vi "Teleop.vi"(10 "Match Info":T1={"Autonomous Elapsed Seconds"=0.0, "TeleOp Elapsed Seconds"=0.0, "Disabled Elapsed Seconds"=0.0, "Visited Autonomous"=FALSE, "Visited TeleOp"=FALSE, "Visited Disabled"=FALSE, "Autonomous Settings"={"Autonomous Style"=enum."Independent", "VI Refnum"=refnum}}, 11 "Call Context":T2) -> ()   [LabVIEW 2014]
doc: "This VI is called for each TeleOp packet received from the DS where the robot is not disabled. It is often used to read from the joysticks and update I/O or to update setpoints for timed control loops. It should complete and return within 20 milliseconds or it may miss DS packets."
uses:
  <vilib>/Rock Robotics/WPI/DriverStation/WPI_DriverStationDerivedRobotMode.ctl
  <vilib>/Rock Robotics/WPI/DriverStation/WPI_DriverStationMatch Info.ctl
  <vilib>/Rock Robotics/WPI/Relay/WPI_RelayValue.ctl
  Robot Global Data.vi
  <vilib>/Rock Robotics/WPI/RobotDrive/WPI_RobotDriveGetSetRefNum.vi
  <vilib>/Rock Robotics/WPI/Joystick/WPI_JoystickGetSetRefNum.vi
  <vilib>/Rock Robotics/WPI/Solenoid/WPI_SolenoidValue.ctl
  <vilib>/Rock Robotics/WPI/Solenoid/WPI_SolenoidSetEnum.vi
panel:
  out "Numeric 1":dbl(slide) scale=0.0..100.0
  out "Boolean 2":bool
  out "Boolean 1":bool
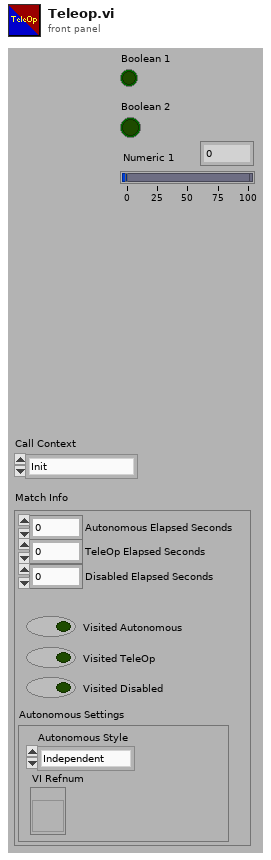
[diagram p1: front panel]
types:
  T1 = typedef "WPI_DriverStationMatch Info.ctl" = cluster{"Autonomous Elapsed Seconds":dbl, "TeleOp Elapsed Seconds":dbl, "Disabled Elapsed Seconds":dbl, "Visited Autonomous":bool, "Visited TeleOp":bool, "Visited Disabled":bool, "Autonomous Settings":cluster{"Autonomous Style":enum16{"Iterative", "Independent"}, "VI Refnum":refnum<vi>}}
  T2 = typedef "WPI_DriverStationDerivedRobotMode.ctl" = enum16{"Init", "Execute", "Stop"}
  T3 = typedef "WPI_RobotDriveDevRef.ctl" = cluster{"DevStatus":errorcluster, "Motors[]":T4[], "Square Inputs":bool, "Max Output":dbl}
  T4 = typedef "WPI_MotorControlDeviceRef.ctl" = cluster{"DeviceStatus":errorcluster, "Type":enum16{"PWM", "CAN"}, "PWM":cluster{"Digital Module":T5, "PWM Channel":T6, "DeadBand":T7}, "CAN":cluster{"Device Number":u8, "Control Mode":T8, "Semaphore":T9, "Max Vout":dbl}, "Invert":bool, "TransformRef":T10, "InvTransformRef":T10}
  T5 = typedef "FPGA_TypedefDigitalModule.ctl" = enum16{"Digital Module 1", "Digital Module 2"}
  T6 = typedef "FPGA_DIOPWMChannel.ctl" = enum8{"PWM 1", "PWM 2", "PWM 3", "PWM 4", "PWM 5", "PWM 6", "PWM 7", "PWM 8", "PWM 9", "PWM 10", "Invalid"}
  T7 = typedef "WPI_PWMDeadband.ctl" = cluster{"Name":string, "maxPositivePwm":i32, "minPositivePwm":i32, "centerPwm":i32, "maxNegativePwm":i32, "minNegativePwm":i32, "angularRange":u16}
  T8 = typedef "WPI_CANJaguar_ControlMode.ctl" = enum8{"Percent VBus", "Current", "Speed", "Position", "Voltage"}
  T9 = typedef "Semaphore RefNum" = refnum<k1>
  T10 = typedef "WPI_PWMTransform_ConPane.ctl" = refnum<vi>
  T11 = typedef "WPI_JoystickDevRef.ctl" = cluster{"Device":T12}
  T12 = typedef "WPI_JoystickDeviceEnum.ctl" = enum16{"USB 0", "USB 1", "USB 2", "USB 3", "USB 4", "USB 5"}
  T13 = cluster{"Button 1":bool, "Button 2":bool, "Button 3":bool, "Button 4":bool, "Button 5":bool, "Button 6":bool, "Button 7":bool, "Button 8":bool, "Button 9":bool, "Button 10":bool, "Button 11":bool, "Button 12":bool}
  T14 = cluster{"axis 1 (x)":dbl, "axis 2 (y)":dbl, "axis 3 (throttle)":dbl, "axis 4":dbl, "axis 5":dbl, "axis 6":dbl}
  T15 = typedef "WPI_DigitalOutputDevRef.ctl" = cluster{"Digital Module":T5, "DIO Channel":T16, "DevStatus":errorcluster}
  T16 = typedef "FPGA_DIOChannel.ctl" = enum8{"DIO 1", "DIO 2", "DIO 3", "DIO 4", "DIO 5", "DIO 6", "DIO 7", "DIO 8", "DIO 9", "DIO 10", "DIO 11", "DIO 12", "DIO 13", "DIO 14", "Invalid"}
  T17 = typedef "WPI_DigitalInputDevRef.ctl" = cluster{"DevStatus":errorcluster, "DIO Channel":T16, "Digital Module":T5}
  T18 = typedef "WPI_SolenoidValue.ctl" = enum16{"Off", "On", "Forward", "Reverse"}
  T19 = typedef "WPI_SolenoidDevRef.ctl" = cluster{"DevStatus":errorcluster, "Solenoid Module":T20, "Forward Solenoid Channel":T21, "Reverse Solenoid Channel":T21}
  T20 = typedef "FPGA_TypedefSolenoidModule.ctl" = enum16{"Solenoid Module 1", "Solenoid Module 2"}
  T21 = typedef "WPI_SolenoidChannel.ctl" = enum8{"Solenoid 1", "Solenoid 2", "Solenoid 3", "Solenoid 4", "Solenoid 5", "Solenoid 6", "Solenoid 7", "Solenoid 8", "Invalid"}
  T22 = typedef "WPI_RelayDevRef.ctl" = cluster{"DevStatus":errorcluster, "Relay Channel":T23, "Digital Module":T5, "Relay Direction":T24}
  T23 = typedef "FPGA_DIORelayChannel.ctl" = enum8{"Relay 1", "Relay 2", "Relay 3", "Relay 4", "Relay 5", "Relay 6", "Relay 7", "Relay 8", "Invalid"}
  T24 = typedef "WPI_RelayDirection.ctl" = enum16{"Both directions", "Forward only", "Reverse only"}
  T25 = typedef "WPI_RelayValue.ctl" = enum16{"Off", "On", "Forward", "Reverse"}
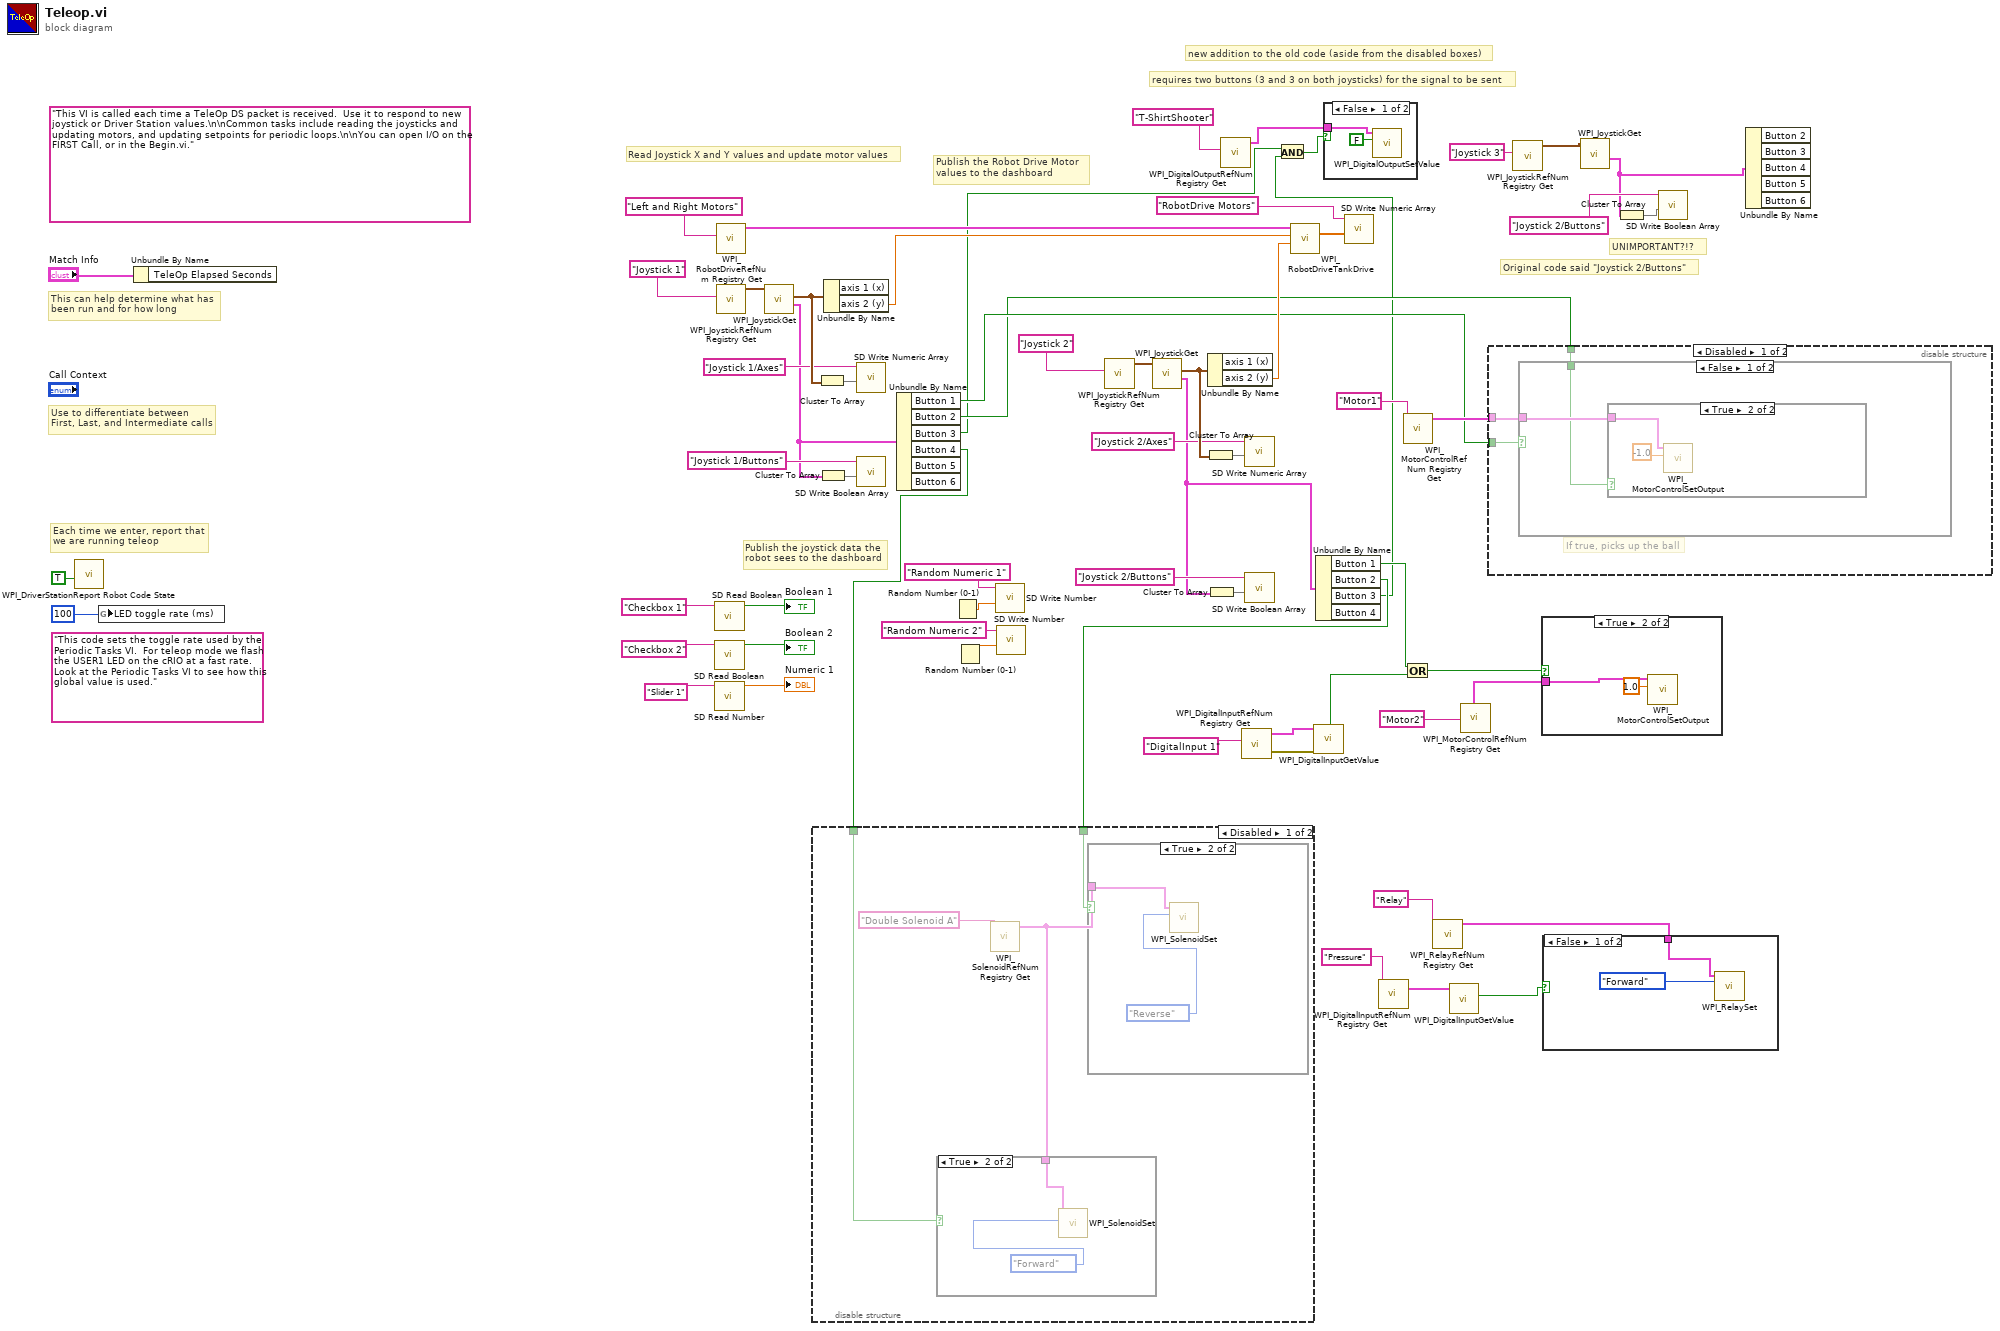
[diagram p0: block diagram]
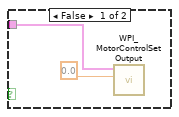
[diagram p2: hidden frame]
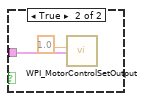
[diagram p3: hidden frame]
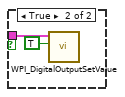
[diagram p8: hidden frame]
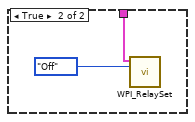
[diagram p9: hidden frame]
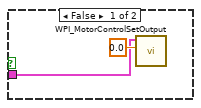
[diagram p10: hidden frame]
diagram:
  (unwired) "This code sets the toggle rate used by the Periodic Tasks VI.  For teleop mode we flash the USER1 LED on the cRIO at a fast rate.  Look at the Periodic Tasks VI to see how this global value is used."
  (unwired) "This VI is called each time a TeleOp DS packet is received.  Use it to respond to new joystick or Driver Station values.\n\nCommon tasks include reading the joysticks and updating motors, and updating setpoints for periodic loops.\n\nYou can open I/O on the FIRST Call, or in the Begin.vi."
  # "Original code said \"Joystick 2/Buttons\""
  # "UNIMPORTANT?!?"
  # "new addition to the old code (aside from the disabled boxes)"
  # "requires two buttons (3 and 3 on both joysticks) for the signal to be sent"
  # "Publish the Robot Drive Motor\nvalues to the dashboard"
  # "Publish the joystick data the\nrobot sees to the dashboard"
  # "Read Joystick X and Y values and update motor values"
  # "Each time we enter, report that\nwe are running teleop"
  # "Use to differentiate between\nFirst, Last, and Intermediate calls"
  # "This can help determine what has\nbeen run and for how long"
  n1 = call <vilib>:"WPI_DriverStationReport Robot Code State.vi"("TeleOp"=TRUE ("Autonomous")) -> ()  [unwired: 10 in, 1 out]
  n2 = global write "Robot Global Data.vi" "LED toggle rate (ms)"(u32 100 ("LED ms toggle rate")) -> ()
  n3 = Unbundle By Name("Match Info") -> ()  [unwired: 1 out]
  n4 = call <vilib>:"SD Read Boolean.vi"("Name"="Checkbox 1" ("refnum name")) -> ("Boolean"=→"Boolean 1":bool)  [unwired: 8 in, 2 out]
  n5 = call <vilib>:"SD Read Boolean.vi"("Name"="Checkbox 2" ("refnum name")) -> ("Boolean"=→"Boolean 2":bool)  [unwired: 8 in, 2 out]
  n6 = call <vilib>:"SD Read Number.vi"("Name"="Slider 1" ("refnum name")) -> ("Numeric"=→"Numeric 1":dbl)  [unwired: 8 in, 2 out]
  n7 = call <vilib>:"WPI_RobotDriveRefNum Registry Get.vi"("refnum name"="Left and Right Motors") -> ("RobotDriveDevRef"=w54:T3)  [unwired: 1 in, 9 out]
  n8 = call <vilib>:"WPI_JoystickRefNum Registry Get.vi"("refnum name"="Joystick 1") -> ("JoystickDevRef"=w52:T11)  [unwired: 1 in, 9 out]
  n9 = call <vilib>:"WPI_JoystickGet.vi"("JoystickDevRef"=w52) -> ("Buttons"=w27:T13, "Axes"=w49:T14)  [unwired: 1 in, 4 out]
  n10 = Cluster To Array(cluster=w49) -> (array=w48:dbl[])
  n11 = Cluster To Array(cluster=w27) -> (array=w51:bool[])
  n12 = Unbundle By Name(w49) -> ("axis 2 (y)"=w32:dbl)  [unwired: 1 out]
  n13 = call <vilib>:"SD Write Numeric Array.vi"("Numeric Array"=w48, "Name"="Joystick 1/Axes") -> ()  [unwired: 8 in, 2 out]
  n14 = call <vilib>:"SD Write Boolean Array.vi"("Boolean Array"=w51, "Name"="Joystick 1/Buttons") -> ()  [unwired: 8 in, 2 out]
  n15 = Unbundle By Name(w27) -> ("Button 1"=w8:bool, "Button 2"=w7:bool, "Button 3"=w3:bool, "Button 4"=w2:bool)  [unwired: 2 out]
  n16 = Random Number (0-1)() -> (number: 0 to 1=w44:dbl)
  n17 = Random Number (0-1)() -> (number: 0 to 1=w43:dbl)
  n18 = call <vilib>:"SD Write Number.vi"("Numeric"=w44, "Name"="Random Numeric 1") -> ()  [unwired: 8 in, 2 out]
  n19 = call <vilib>:"SD Write Number.vi"("Numeric"=w43, "Name"="Random Numeric 2") -> ()  [unwired: 8 in, 2 out]
  n20 = call <vilib>:"WPI_JoystickRefNum Registry Get.vi"("refnum name"="Joystick 2") -> ("JoystickDevRef"=w39:T11)  [unwired: 1 in, 9 out]
  n21 = call <vilib>:"WPI_JoystickGet.vi"("JoystickDevRef"=w39) -> ("Buttons"=w28:T13, "Axes"=w36:T14)  [unwired: 1 in, 4 out]
  n22 = Cluster To Array(cluster=w36) -> (array=w35:dbl[])
  n23 = Cluster To Array(cluster=w28) -> (array=w38:bool[])
  n24 = Unbundle By Name(w36) -> ("axis 2 (y)"=w20:dbl)  [unwired: 1 out]
  n25 = call <vilib>:"WPI_DigitalOutputRefNum Registry Get.vi"("refnum name"="T-ShirtShooter") -> ("DigitalOutputDevRef"=w5:T15)  [unwired: 9 in, 1 out]
  n26 = call <vilib>:"WPI_DigitalInputRefNum Registry Get.vi"("refnum name"="DigitalInput 1") -> ("error out"=w29:errorcluster, "DigitalInputDevRef"=w30:T17)  [unwired: 9 in]
  n27 = call <vilib>:"SD Write Numeric Array.vi"("Numeric Array"=w35, "Name"="Joystick 2/Axes") -> ()  [unwired: 8 in, 2 out]
  n28 = call <vilib>:"SD Write Boolean Array.vi"("Boolean Array"=w38, "Name"="Joystick 2/Buttons") -> ()  [unwired: 8 in, 2 out]
  n29 = call <vilib>:"WPI_RobotDriveTankDrive.vi"("Right axis value"=w20, "Left axis value"=w32, "RobotDriveDevRef"=w54) -> ("Motor Values"=w45:dbl[])  [unwired: 6 in, 2 out]
  n30 = call <vilib>:"WPI_DigitalInputGetValue.vi"("error in (no error)"=w29, "DigitalInputDevRef"=w30) -> ("Value"=w24:bool)  [unwired: 7 in, 2 out]
  n31 = Unbundle By Name(w28) -> ("Button 1"=w10:bool, "Button 2"=w9:bool, "Button 3"=w1:bool)  [unwired: 1 out]
  n32 = disable-structure shown="Disabled" {
    disable-tunnel: w9 -> [w66 _]
    disable-tunnel: w2 -> [w65 _]
    frame Disabled {
      n33 = call <vilib>:"WPI_SolenoidRefNum Registry Get.vi"("refnum name"="Double Solenoid A") -> ("SolenoidDevRef"=w67:T19)  [unwired: 9 in, 1 out]
      n34 = case shown="True" w65 {
        tunnel: w67 -> [_ w71]
        frame False {
        }
        frame True {
          n35 = call-poly <vilib>:"WPI_SolenoidSet.vi"("Value"=WPI_SolenoidValue."Forward", "SolenoidDevRef"=w71) -> ()  [unwired: 8 in, 2 out]
        }
      }
      n36 = case shown="True" w66 {
        tunnel: w67 -> [_ w70]
        frame False {
        }
        frame True {
          n37 = call-poly <vilib>:"WPI_SolenoidSet.vi"("Value"=WPI_SolenoidValue."Reverse" ("f"), "SolenoidDevRef"=w70) -> ()  [unwired: 8 in, 2 out]
        }
      }
    }
    frame Enabled {
    }
  }
  n38 = And(x=w3, y=w1) -> (x .and. y?=w4:bool)
  n39 = case shown="False" w4 {
    tunnel: w5 -> [w73 w76]
    frame False {
      n40 = call <vilib>:"WPI_DigitalOutputSetValue.vi"("Value"=FALSE, "DigitalOutputDevRef"=w73) -> ()  [unwired: 8 in, 2 out]
    }
    frame True {
      n41 = call <vilib>:"WPI_DigitalOutputSetValue.vi"("Value"=TRUE, "DigitalOutputDevRef"=w76) -> ()  [unwired: 8 in, 2 out]
    }
  }
  n42 = call <vilib>:"SD Write Numeric Array.vi"("Numeric Array"=w45, "Name"="RobotDrive Motors") -> ()  [unwired: 8 in, 2 out]
  n43 = call <vilib>:"WPI_DigitalInputRefNum Registry Get.vi"("refnum name"="Pressure") -> ("DigitalInputDevRef"=w21:T17)  [unwired: 9 in, 1 out]
  n44 = Or(x=w10, y=w24) -> (x .or. y?=w23:bool)
  n45 = call <vilib>:"WPI_MotorControlRefNum Registry Get.vi"("refnum name"="Motor1") -> ("MotorControlDevRef"=w11:T4)  [unwired: 9 in, 1 out]
  n46 = call <vilib>:"WPI_RelayRefNum Registry Get.vi"("refnum name"="Relay") -> ("RelayDevRef"=w22:T22)  [unwired: 9 in, 1 out]
  n47 = call <vilib>:"WPI_DigitalInputGetValue.vi"("DigitalInputDevRef"=w21) -> ("Value"=w17:bool)  [unwired: 8 in, 2 out]
  n48 = call <vilib>:"WPI_MotorControlRefNum Registry Get.vi"("refnum name"="Motor2") -> ("MotorControlDevRef"=w25:T4)  [unwired: 9 in, 1 out]
  n49 = disable-structure shown="Disabled" {
    disable-tunnel: w11 -> [w79 _]
    disable-tunnel: w8 -> [w78 _]
    disable-tunnel: w7 -> [w77 _]
    frame Disabled {
      # "If true, picks up the ball"
      n50 = case shown="False" w78 {
        tunnel: w79 -> [w81 w87]
        tunnel: w77 -> [w80 _]
        frame False {
          n51 = case shown="True" w80 {
            tunnel: w81 -> [w82 w84]
            frame False {
              n52 = call <vilib>:"WPI_MotorControlSetOutput.vi"("Output"=0.0, "MotorControlDevRef"=w82) -> ()  [unwired: 7 in, 3 out]
            }
            frame True {
              n53 = call <vilib>:"WPI_MotorControlSetOutput.vi"("Output"=-1.0, "MotorControlDevRef"=w84) -> ()  [unwired: 7 in, 3 out]
            }
          }
        }
        frame True {
          n54 = call <vilib>:"WPI_MotorControlSetOutput.vi"("Output"=1.0, "MotorControlDevRef"=w87) -> ()  [unwired: 7 in, 3 out]
        }
      }
    }
    frame Enabled {
    }
  }
  n55 = call <vilib>:"WPI_JoystickRefNum Registry Get.vi"("refnum name"="Joystick 3") -> ("JoystickDevRef"=w15:T11)  [unwired: 9 in, 1 out]
  n56 = case shown="True" w23 {
    tunnel: w25 -> [w88 w91]
    frame False {
      n57 = call <vilib>:"WPI_MotorControlSetOutput.vi"("Output"=0.0, "MotorControlDevRef"=w88) -> ()  [unwired: 7 in, 3 out]
    }
    frame True {
      n58 = call <vilib>:"WPI_MotorControlSetOutput.vi"("Output"=1.0, "MotorControlDevRef"=w91) -> ()  [unwired: 7 in, 3 out]
    }
  }
  n59 = case shown="False" w17 {
    tunnel: w22 -> [w92 w94]
    frame False {
      n60 = call <vilib>:"WPI_RelaySet.vi"("RelayValue"=WPI_RelayValue."Forward", "RelayDevRef"=w92) -> ()  [unwired: 8 in, 2 out]
    }
    frame True {
      n61 = call <vilib>:"WPI_RelaySet.vi"("RelayValue"=WPI_RelayValue."Off", "RelayDevRef"=w94) -> ()  [unwired: 8 in, 2 out]
    }
  }
  n62 = call <vilib>:"WPI_JoystickGet.vi"("JoystickDevRef"=w15) -> ("Buttons"=w12:T13)  [unwired: 4 in, 2 out]
  n63 = Cluster To Array(cluster=w12) -> (array=w13:bool[])
  n64 = call <vilib>:"SD Write Boolean Array.vi"("Boolean Array"=w13, "Name"="Joystick 2/Buttons") -> ()  [unwired: 8 in, 2 out]
  n65 = Unbundle By Name(w12) -> ()  [unwired: 5 out]
